vi "例题7.1.vi"() -> ()   [LabVIEW 2017]
panel:
  out "7（X0=10,dx=2，Y）多条曲线":cluster{i32, i32, cluster{dbl[]}[]}(graph)
  out "6（X0=10,dx=2，Y）多条曲线":cluster{i32, i32, dbl[][]}(graph)
  out "5（X0=10,dx=2，Y）多条曲线":cluster{i32, i32, dbl[]}[](graph)
  out "4（X0=10,dx=2，Y）单条曲线":cluster{i32, i32, dbl[]}(graph)
  out "3（Y）多条曲线 2":cluster{dbl[]}[](graph)
  out "2（Y）多条曲线":dbl[][](graph)
  out "1（Y）单条曲线":dbl[](graph)
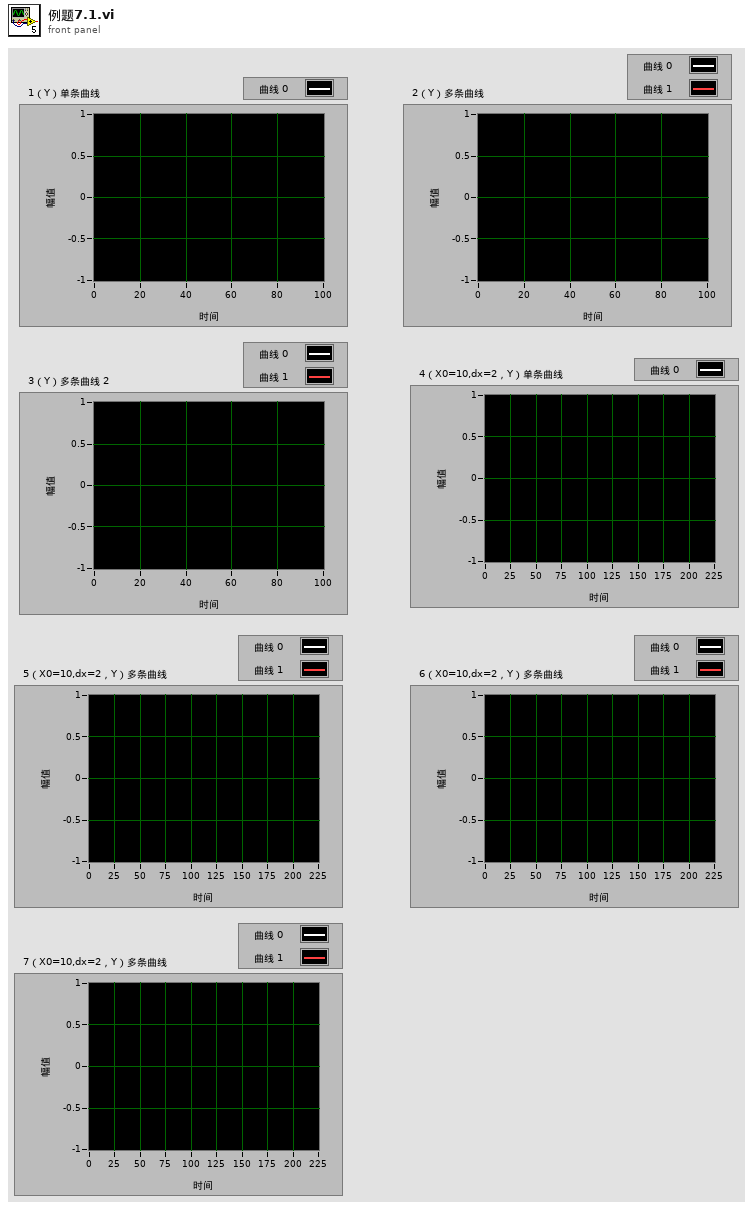
[diagram p1: front panel]
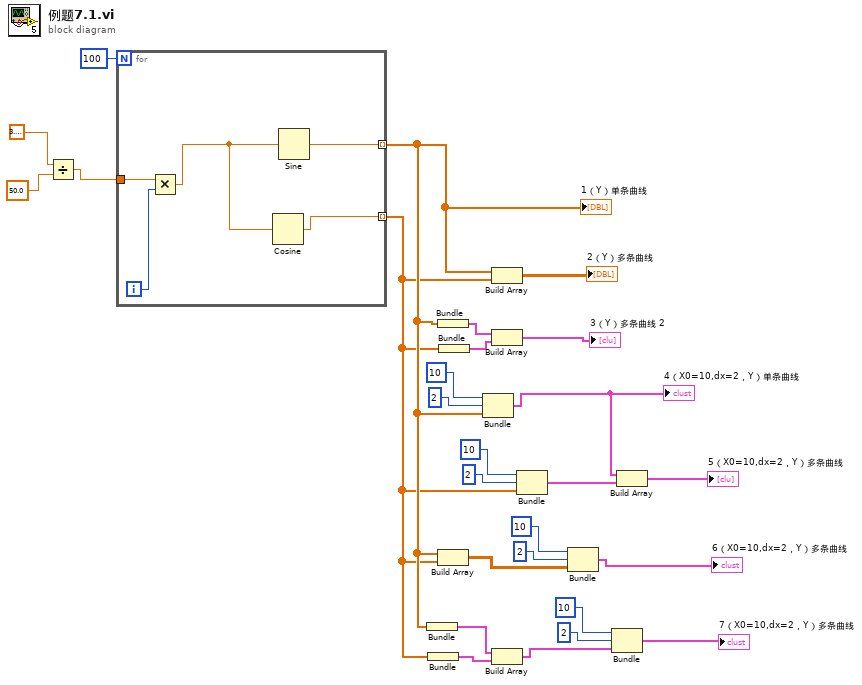
[diagram p0: block diagram]
diagram:
  n1 = Divide(x=3.141592653589793, y=50.0) -> (x/y=w24:dbl)
  n2 = for {
    N: 100 -> [_]
    tunnel: w24 -> [w32]
    tunnel: [w29] -> w10 mode=indexing
    tunnel: [w28] -> w9 mode=indexing
    i -> [w31]
    n3 = Multiply(x=w32, y=w31) -> (x*y=w30:dbl)
    n4 = Cosine(x=w30) -> (cos(x)=w28:dbl)
    n5 = Sine(x=w30) -> (sin(x)=w29:dbl)
  }
  "1（Y）单条曲线" <- w10
  n6 = Bundle(w10) -> (w8:cluster{dbl[]})  [unwired: 1 in]
  n7 = Bundle(w9) -> (w7:cluster{dbl[]})  [unwired: 1 in]
  n8 = Bundle(w10) -> (w22:cluster{dbl[]})  [unwired: 1 in]
  n9 = Build Array(w10, w9) -> (w11:dbl[][])
  n10 = Bundle(w9) -> (w21:cluster{dbl[]})  [unwired: 1 in]
  n11 = Bundle(10, 2, w10) -> (w4:cluster{i32, i32, dbl[]})  [unwired: 1 in]
  "4（X0=10,dx=2，Y）单条曲线" <- w4
  n12 = Build Array(w10, w9) -> (→"2（Y）多条曲线":dbl[][])
  n13 = Build Array(w22, w21) -> (→"3（Y）多条曲线 2":cluster{dbl[]}[])
  n14 = Build Array(w8, w7) -> (w6:cluster{dbl[]}[])
  n15 = Bundle(10, 2, w9) -> (w5:cluster{i32, i32, dbl[]})  [unwired: 1 in]
  n16 = Bundle(10, 2, w11) -> (→"6（X0=10,dx=2，Y）多条曲线":cluster{i32, i32, dbl[][]})  [unwired: 1 in]
  n17 = Bundle(10, 2, w6) -> (→"7（X0=10,dx=2，Y）多条曲线":cluster{i32, i32, cluster{dbl[]}[]})  [unwired: 1 in]
  n18 = Build Array(w4, w5) -> (→"5（X0=10,dx=2，Y）多条曲线":cluster{i32, i32, dbl[]}[])
